vi "RandomizeBackground.vi"(7 "Possibility":dbl=0.5 format="%#_13g", 8 "error in (no error)":errorcluster, 9 "ReplaceTilecode":u8=255, 10 "ToReplaceTilecode":u8, 11 "Menu in":refnum<class "Menu.lvclass">) -> (0 "error out":errorcluster, 3 "Menu out":refnum<class "Menu.lvclass">)   [LabVIEW 2019, in "RT_Game.lvlib" / "Menu.lvclass"]
uses:
  Menu.lvclass
  C:/Users/FreshBob/Dropbox/VIs/myRIO_GameConsole/RT/RT_Game/Game/Game.lvclass
  Game/Game.lvclass/Game.ctl
  Game/Read Tiles.vi
  Game/Write Tiles.vi
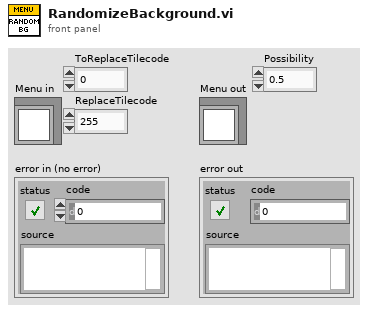
[diagram p1: front panel]
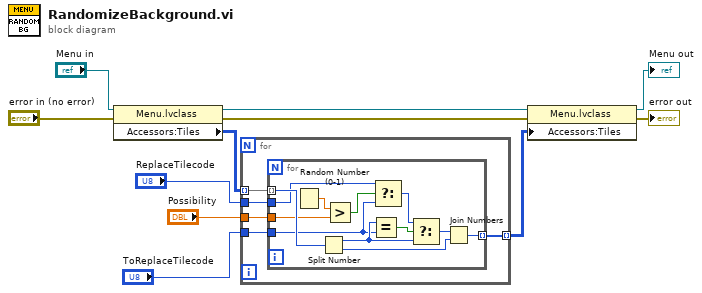
[diagram p0: block diagram]
diagram:
  n1 = property class="Menu.lvclass"(reference="Menu in", error in="error in (no error)") -> (reference out=w8:refnum<class "Menu.lvclass">, error out=w5:errorcluster, "Accessors:Tiles"=w10:u16[][])
  n2 = for {
    tunnel: w10 -> [w16] mode=indexing
    tunnel: [w15] -> w11 mode=indexing
    tunnel: "ToReplaceTilecode" -> [w14]
    tunnel: "ReplaceTilecode" -> [w13]
    tunnel: "Possibility" -> [w12]
    n3 = for {
      tunnel: w16 -> [w28] mode=indexing
      tunnel: [w21] -> w15 mode=indexing
      tunnel: w14 -> [w19]
      tunnel: w13 -> [w18]
      tunnel: w12 -> [w17]
      n4 = Random Number (0-1)() -> (number: 0 to 1=w23:dbl)
      n5 = Split Number(x=w28) -> (hi(x)=w20:u8, lo(x)=w27:u8)
      n6 = Greater?(x=w23, y=w17) -> (0:w22:bool)
      n7 = Equal?(x=w20, y=w19) -> (x = y?=w25:bool)
      n8 = Select(t=w18, s=w22, f=w19) -> (s? t:f=w24:u8)
      n9 = Select(t=w24, s=w25, f=w20) -> (s? t:f=w26:u8)
      n10 = Join Numbers(hi=w26, lo=w27) -> ((hi.lo)=w21:u16)
    }
  }
  n11 = property class="Menu.lvclass"(reference=w8, error in=w5, "Accessors:Tiles"=w11) -> (reference out=→"Menu out":refnum<class "Menu.lvclass">, error out=→"error out":errorcluster)
